vi "ApplySystemDefinitionOverride.vi"(8 "error in (no error)":errorcluster, 10 "override item":T1, 11 "node in":refnum<k20>) -> (0 "error out":errorcluster, 3 "node out":refnum<k20>)   [LabVIEW 2015, in "VeriStandTestUtilities.lvlib"]
uses:
  VeriStandTestUtilities.lvlib
  <vilib>/xml/NI_XML.lvlib
  <resource>/objmgr/DOMUserDefRef.rc
  <vilib>/httpClient/LabVIEWHTTPClient.lvlib
panel:
  in  "No matches error":string="No matches were found for the following override string: "
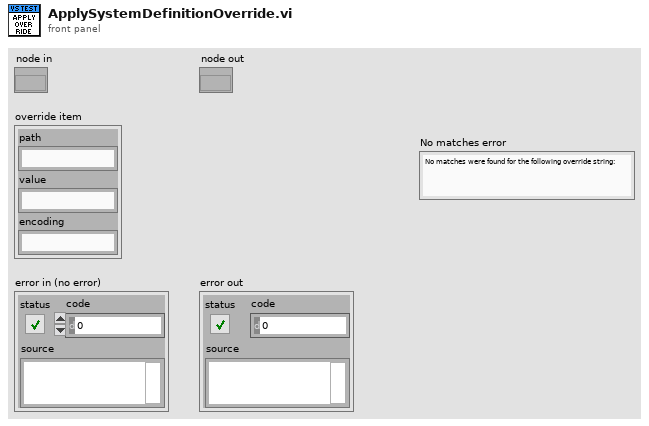
[diagram p1: front panel]
types:
  T1 = cluster{"path":string, "value":string, "encoding":string}
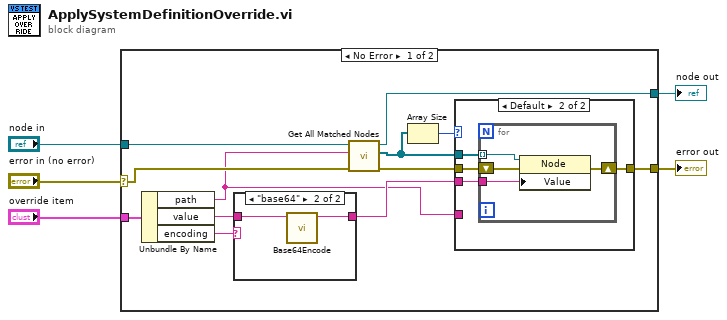
[diagram p0: block diagram]
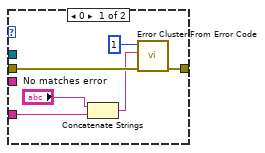
[diagram p2: hidden frame]
diagram:
  n1 = case shown="No Error" "error in (no error)" {
    selector: "error in (no error)" -> [w13 w36]
    tunnel: "override item" -> [w17 _]
    tunnel: [w16 w36] -> w4
    tunnel: [w14 w35] -> w3
    tunnel: "node in" -> [w12 w35]
    frame No Error {
      n2 = Unbundle By Name(w17) -> ("path"=w6:string, "value"=w10:string, "encoding"=w11:string)
      n3 = case shown="\"base64\"" w11 {
        tunnel: [w32 w34] -> w9
        tunnel: w10 -> [w32 w33]
        frame Default {
        }
        frame "base64" {
          n4 = call <vilib>:"Base64Encode.vi"("buffer in"=w33) -> ("encoded string"=w34:string)  [unwired: 9 in, 1 out]
        }
      }
      n5 = call <vilib>:"Get All Matched Nodes.vi"("error in (no error)"=w13, "XPath expression"=w6, "node in"=w12) -> ("error out"=w15:errorcluster, "node result array"=w8:refnum<k20>[], "node out"=w14:refnum<k20>)  [unwired: 6 in]
      n6 = Array Size(array=w8) -> (size(s)=w7:i32)
      n7 = case shown="Default" w7 {
        tunnel: [w22 w27] -> w16
        tunnel: w15 -> [w23 w26]
        tunnel: w9 -> [_ w25]
        tunnel: w8 -> [_ w24]
        tunnel: w6 -> [w18 _]
        frame 0 {
          n8 = Concatenate Strings("No matches error", w18) -> (w20:string)
          n9 = call <vilib>:"Error Cluster From Error Code.vi"("error in (no error)"=w23, "error message (\"\")"=w20, "error code (0)"=1) -> ("error out"=w22:errorcluster)  [unwired: 6 in]
        }
        frame Default {
          n10 = for {
            shift-right: [w30] -> w27
            shift-left: w26 -> [w31]
            tunnel: w24 -> [w29] mode=indexing
            tunnel: w25 -> [w28]
            n11 = property class="Node"(reference=w29, error in=w31, "Value"=w28) -> (error out=w30:errorcluster)  [unwired: 1 out]
          }
        }
      }
    }
    frame Error {
    }
  }
  "error out" <- w4
  "node out" <- w3
